vi "bfield_ellipse.vi"(8 "phi":dbl[](array[numeric]), 11 "parameters":T1) -> (3 "B(a,phi) as 1D":dbl[](array[numeric]))   [LabVIEW 2017]
uses:
  typedefs/magnetic field fit.ctl
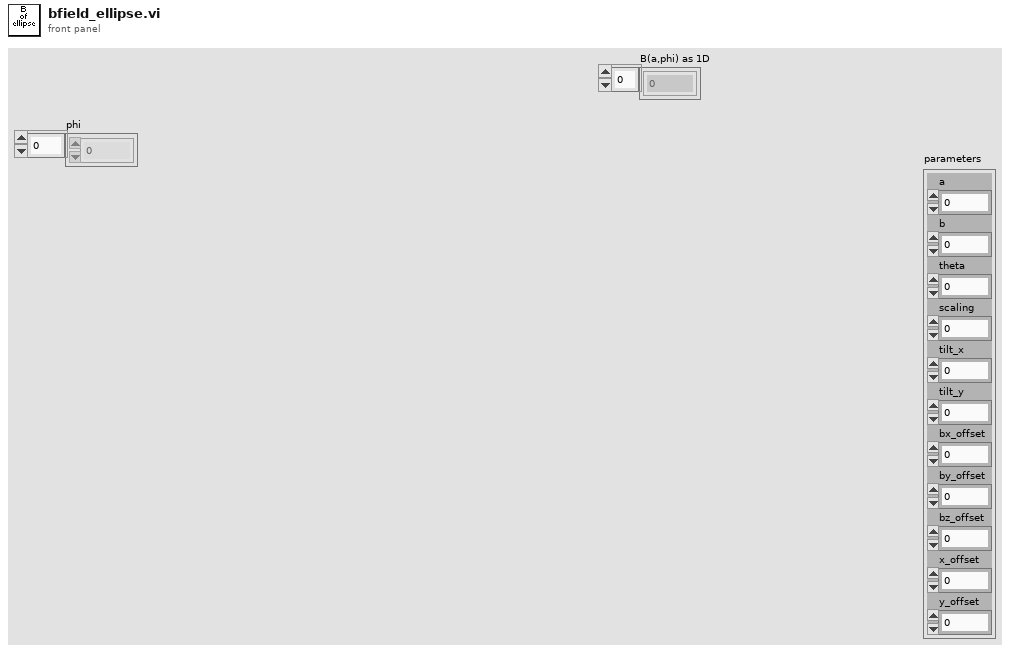
[diagram p1: front panel]
types:
  T1 = typedef "magnetic field fit.ctl" = cluster{"a":dbl, "b":dbl, "theta":dbl, "scaling":dbl, "tilt_x":dbl, "tilt_y":dbl, "bx_offset":dbl, "by_offset":dbl, "bz_offset":dbl, "x_offset":dbl, "y_offset":dbl}
  T2 = cluster{"bx_offset":dbl, "by_offset":dbl, "bz_offset":dbl}
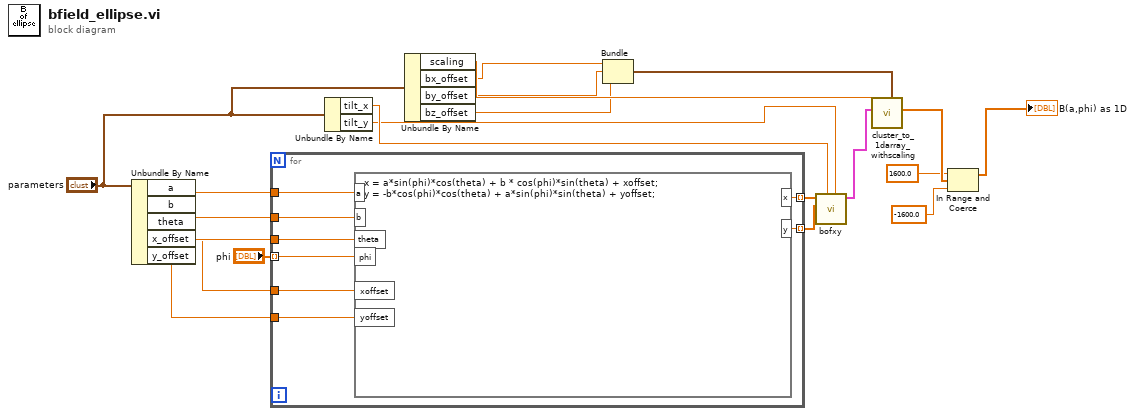
[diagram p0: block diagram]
diagram:
  n1 = Unbundle By Name("parameters") -> ("a"=w18:dbl, "b"=w17:dbl, "theta"=w16:dbl, "x_offset"=w2:dbl, "y_offset"=w1:dbl)
  n2 = for {
    tunnel: "phi" -> [w29] mode=indexing
    tunnel: [w28] -> w20 mode=indexing
    tunnel: [w27] -> w19 mode=indexing
    tunnel: w18 -> [w26]
    tunnel: w17 -> [w25]
    tunnel: w16 -> [w24]
    tunnel: w2 -> [w23]
    tunnel: w1 -> [w22]
    n3 = formula code="x = a*sin(phi)*cos(theta) + b * cos(phi)*sin(theta) + xoffset;\ny = -b*cos(phi)*cos(theta) + a*sin(phi)*sin(theta) + yoffset;"("a"=w26, "b"=w25, "theta"=w24, "phi"=w29, "xoffset"=w23, "yoffset"=w22) -> ("x"=w28:dbl, "y"=w27:dbl)
  }
  n4 = Unbundle By Name("parameters") -> ("tilt_x"=w15:dbl, "tilt_y"=w14:dbl)
  n5 = Unbundle By Name("parameters") -> ("scaling"=w11:dbl, "bx_offset"=w10:dbl, "by_offset"=w9:dbl, "bz_offset"=w8:dbl)
  n6 = Bundle("bx_offset"=w10, "by_offset"=w9, "bz_offset"=w8) -> (w7:T2)  [unwired: 1 in]
  n7 = call "bofxy.vi"("tilt_y"=w14, "tilt_x"=w15, "Y"=w19, "X"=w20) -> ("B"=w13:cluster{"Bx":dbl[], "By":dbl[], "Bz":dbl[]})  [unwired: 5 in, 2 out]
  n8 = call "cluster_to_1darray_withscaling.vi"("Boffset"=w7, "scaling"=w11, "B"=w13) -> ("scaledBarray"=w6:dbl[])  [unwired: 8 in]
  n9 = In Range and Coerce(upper limit=1600.0, x=w6, lower limit=-1600.0) -> (coerced(x)=→"B(a,phi) as 1D":dbl[])  [unwired: 1 out]
